vi "SaveResultFile.vi"(8 "error in (no error)":errorcluster, 10 "FolderPath":path, 11 "CAlexData2 in":refnum<class "CAlexData2.lvclass">) -> (0 "error out":errorcluster, 2 "FilePath":path, 3 "CAlexData2 out":refnum<class "CAlexData2.lvclass">)   [LabVIEW 2015, in "CAlexData2.lvclass"]
uses:
  CAlexData2.lvclass
  <vilib>/Utility/file.llb/Write To Spreadsheet File (DBL).vi
  CustomVIs/CustomVI.lvlib
panel:
  in  "Dilate Length":i32=500
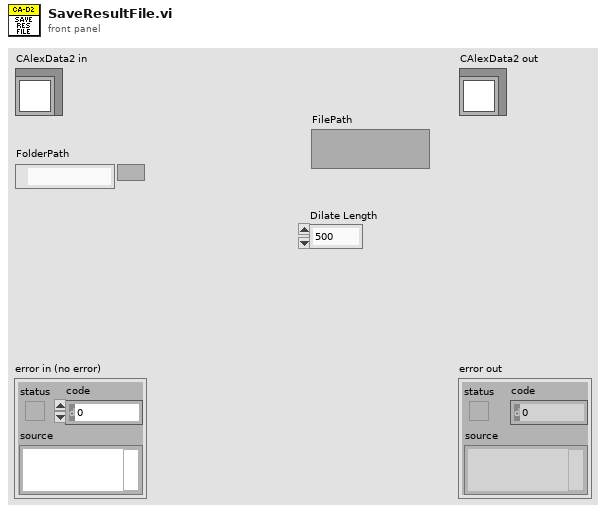
[diagram p1: front panel]
types:
  T1 = enum16{"open", "replace", "create", "open or create", "replace or create", "replace or create with confirmation"}
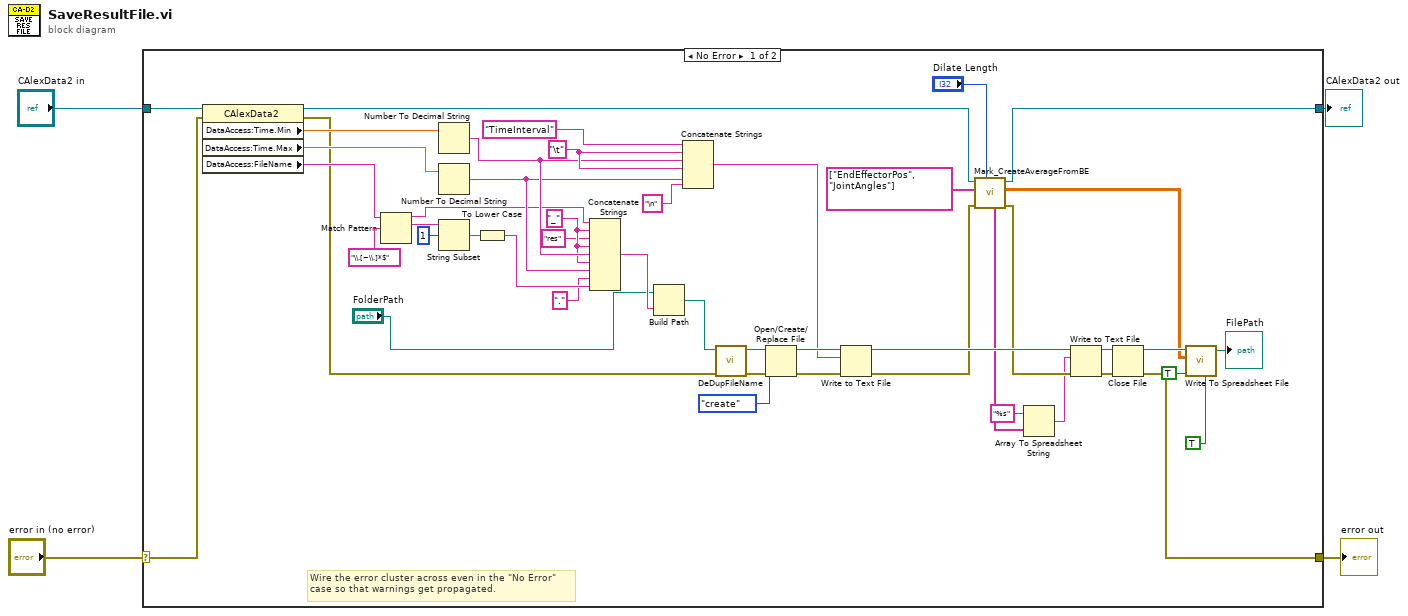
[diagram p0: block diagram]
diagram:
  n1 = case shown="No Error" "error in (no error)" {
    selector: "error in (no error)" -> [w49 w53]
    tunnel: [w25 w53] -> w3
    tunnel: [w39 w52] -> w1
    tunnel: "CAlexData2 in" -> [w50 w52]
    frame No Error {
      w8 = "_" ("string")
      w45 = "\t" ("string")
      # "Wire the error cluster across even in the \"No Error\"\ncase so that warnings get propagated."
      n2 = property class="CAlexData2"(reference=w50, error in=w49) -> (reference out=w40:refnum<class "CAlexData2.lvclass">, error out=w5:errorcluster, "DataAccess:Time.Min"=w48:dbl, "DataAccess:Time.Max"=w47:dbl, "DataAccess:FileName"=w18:string)
      n3 = Match Pattern(string=w18, regular expression="\\.[~\\.]*$") -> (before substring=w9:string, match substring=w19:string)  [unwired: 3 out]
      n4 = Number To Decimal String(number=w48) -> (decimal integer string=w44:string)  [unwired: 1 in]
      n5 = Number To Decimal String(number=w47) -> (decimal integer string=w43:string)  [unwired: 1 in]
      n6 = String Subset(string=w19, offset (0)=1) -> (substring=w20:string)  [unwired: 1 out]
      n7 = To Lower Case(string=w20) -> (all lower case string=w17:string)
      n8 = Concatenate Strings(w9, w8, "res" ("string"), w8, w44, w8, w43, "." ("string"), w17) -> (w42:string)
      n9 = Build Path(base path="FolderPath", name or relative path=w42) -> (appended path=w41:path)
      n10 = Concatenate Strings("TimeInterval", w45, w44, w45, w43, "\n" ("string")) -> (w34:string)
      n11 = call "DeDupFileName.vi"("error in (no error)"=w5, "Path"=w41) -> ("error out"=w37:errorcluster, "Out Path"=w38:path)  [unwired: 7 in, 1 out]
      n12 = Open/Create/Replace File(file path (use dialog)=w38, error in=w37, operation (0:open)=T1."create") -> (refnum out=w35:refnum<file>, error out=w36:errorcluster)  [unwired: 3 in, 1 out]
      n13 = Write to Text File(file (use dialog)=w35, text=w34, error in=w36) -> (refnum out=w29:refnum<file>, error out=w24:errorcluster)  [unwired: 1 in, 1 out]
      n14 = call-dynamic "Mark_CreateAverageFromBE.vi"("Dilate Length"="Dilate Length", "error in (no error)"=w24, "Variables"=string[] ["EndEffectorPos", "JointAngles"], "ExpData in"=w40) -> ("error out"=w23:errorcluster, "Mean"=w31:dbl[][], "ExpData out"=w39:refnum<class "CAlexData2.lvclass">, "ColHeaders"=w14:string[])  [unwired: 3 in, 1 out]
      n15 = Array To Spreadsheet String(array=w14, 3:"%s" ("format string")) -> (spreadsheet string=w13:string)  [unwired: 1 in]
      n16 = Write to Text File(file (use dialog)=w29, text=w13, error in=w23) -> (refnum out=w28:refnum<file>, error out=w27:errorcluster)  [unwired: 1 in, 1 out]
      n17 = Close File(refnum=w28, error in=w27) -> (path=w32:path, error out=w25:errorcluster)
      n18 = call-poly <vilib>:"Write To Spreadsheet File.vi"("transpose? (no:F)"=TRUE, "append to file? (new file:F)"=TRUE, "2D data"=w31, "file path (dialog if empty)"=w32) -> ("new file path (Not A Path if cancelled)"=→"FilePath":path)  [unwired: 4 in]
    }
    frame Error {
    }
  }
  "error out" <- w3
  "CAlexData2 out" <- w1
